vi "Set Origin on Map.vi"(8 "error in (no error)":errorcluster, 10 "Origin on Map":T1, 11 "Map Model in":refnum<class "Map Model.lvclass">) -> (0 "error out":errorcluster, 3 "Map Model out":refnum<class "Map Model.lvclass">)   [LabVIEW 2020, in "Map Model.lvlib" / "Map Model.lvclass"]
uses:
  Map Model.lvclass
  <vilib>/Utility/miscctls.llb/LVPointTypeDef.ctl
  Map Model.lvclass/Map Model.ctl
panel:
  # "NOTICE -- YOU MUST LEAVE THIS NOTICE IN PLACE.\n\nCopyright (c) 2017, LIANG LIU Shawn.Liu.cn@gmail.com\nAll rights reserved.\n\nRedistribution and use in source and binary forms, with or without modification, are permitted provided that the following conditions are met:\n-Redistributions of source code must retain the above copyright notice, this list of conditions and the following disclaimer.\n-Redistributions in binary form must reproduce the above copyright notice, this list of conditions and the following disclaimer in the documentation and/or other materials provided with the distribution.\n-Neither the name of the eLp nor the names of its contributors may be used to endorse or promote products derived from this software without specific prior written permission.\n\nTHIS SOFTWARE IS PROVIDED BY THE COPYRIGHT HOLDERS AND CONTRIBUTORS \"AS IS\" AND ANY EXPRESS OR IMPLIED WARRANTIES, INCLUDING, BUT NOT LIMITED TO, THE IMPLIED WARRANTIES OF MERCHANTABILITY AND FITNESS FOR A PARTICULAR PURPOSE ARE DISCLAIMED. IN NO EVENT SHALL THE COPYRIGHT HOLDER OR CONTRIBUTORS BE LIABLE FOR ANY DIRECT, INDIRECT, INCIDENTAL, SPECIAL, EXEMPLARY, OR CONSEQUENTIAL DAMAGES (INCLUDING, BUT NOT LIMITED TO, PROCUREMENT OF SUBSTITUTE GOODS OR SERVICES; LOSS OF USE, DATA, OR PROFITS; OR BUSINESS INTERRUPTION) HOWEVER CAUSED AND ON ANY THEORY OF LIABILITY, WHETHER IN CONTRACT, STRICT LIABILITY, OR TORT (INCLUDING NEGLIGENCE OR OTHERWISE) ARISING IN ANY WAY OUT OF THE USE OF THIS SOFTWARE, EVEN IF ADVISED OF THE POSSIBILITY OF SUCH DAMAGE."
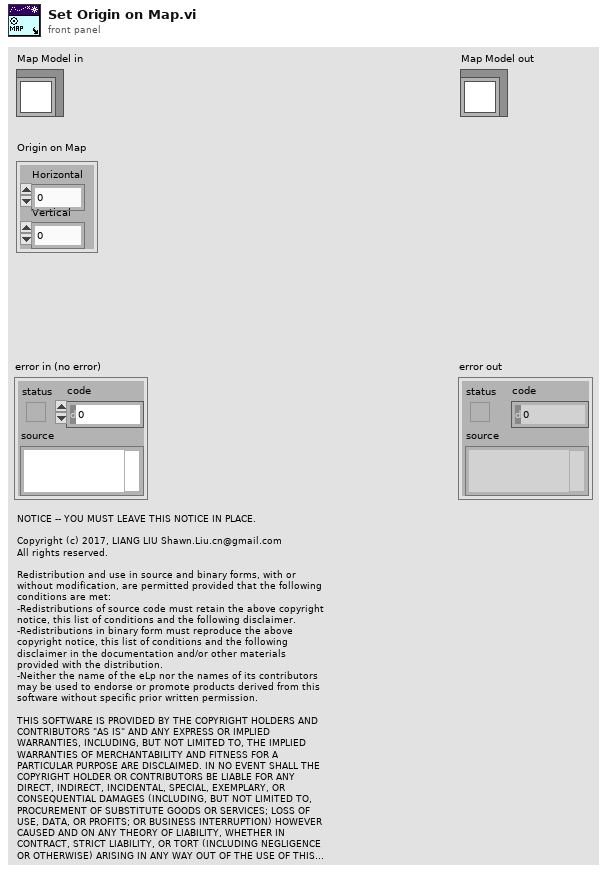
[diagram p1: front panel]
types:
  T1 = typedef "LVPointTypeDef.ctl" = cluster{"Horizontal":i16, "Vertical":i16}
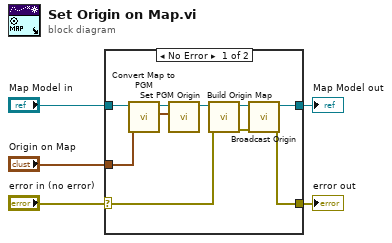
[diagram p0: block diagram]
diagram:
  n1 = case shown="No Error" "error in (no error)" {
    selector: "error in (no error)" -> [w7 w17]
    tunnel: "Map Model in" -> [w15 w16]
    tunnel: [w14 w16] -> w4
    tunnel: "Origin on Map" -> [w8 _]
    tunnel: [w6 w17] -> w1
    frame No Error {
      n2 = call "Convert Map to PGM.vi"("Position on Map"=w8, "Map Model in"=w15) -> ("Position on PGM"=w11:T1, "Map Model out"=w13:refnum<class "Map Model.lvclass">)  [unwired: 8 in]
      n3 = call "Set PGM Origin.vi"("PGM Origin"=w11, "Map Model in"=w13) -> ("Map Model out"=w12:refnum<class "Map Model.lvclass">)  [unwired: 9 in]
      n4 = call "Build Origin Map.vi"("error in (no error)"=w7, "Map Model in"=w12) -> ("error out"=w9:errorcluster, "Map Model out"=w10:refnum<class "Map Model.lvclass">)  [unwired: 8 in]
      n5 = call "Broadcast Origin.vi"("error in (no error)"=w9, "Map Model in"=w10) -> ("error out"=w6:errorcluster, "Map Model out"=w14:refnum<class "Map Model.lvclass">)  [unwired: 8 in]
    }
    frame Error {
    }
  }
  "error out" <- w1
  "Map Model out" <- w4
